vi "Send Message.vi"(8 "error in (no error)":errorcluster, 10 "Message":string, 11 "EUI Events in":refnum<class "EUI Events.lvclass">) -> (0 "error out":errorcluster, 3 "EUI Events out":refnum<class "EUI Events.lvclass">)   [LabVIEW 2016, in "EUI Events.lvclass"]
uses:
  EUI Events.lvclass
  Typedefs/MessageContainer.ctl
  Typedefs/M1M3SupportEUI_TypeDefs.lvlib
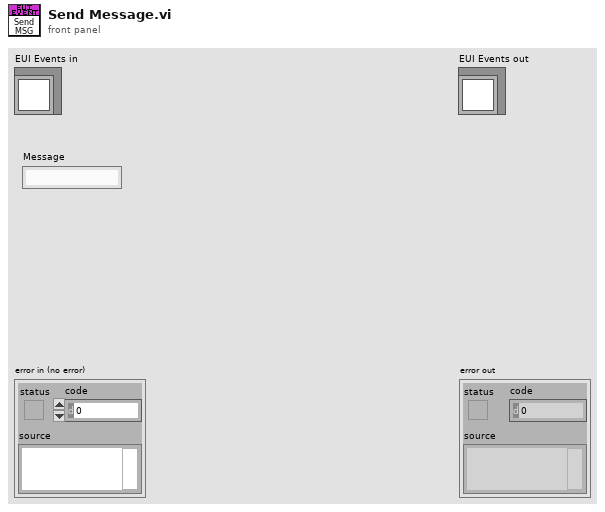
[diagram p1: front panel]
types:
  T1 = typedef "M1M3SupportEUI_TypeDefs.lvlib/MessageContainer.ctl" = cluster{"Message":string, "Time Stamp":timestamp, "Priority":enum16{"Message", "Warning", "Fault", ""}}
  T2 = typedef "M1M3SupportEUI_TypeDefs.lvlib/EUI Events.ctl" = cluster{"Message Event":refnum<user-event>}
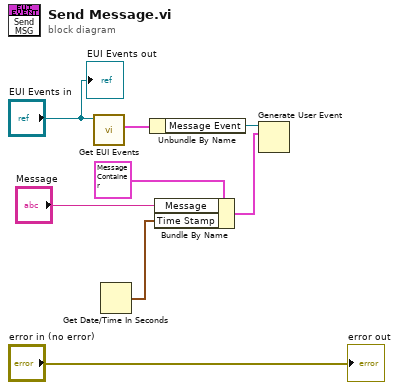
[diagram p0: block diagram]
diagram:
  n1 = call "Get EUI Events.vi"("EUI Events in"="EUI Events in") -> ("EUI Events"=w7:T2)  [unwired: 8 in, 2 out]
  n2 = Get Date/Time In Seconds() -> (seconds since 1Jan1904=w2:timestamp)
  n3 = Unbundle By Name(w7) -> ("Message Event"=w4:refnum<user-event>)
  n4 = Bundle By Name(cluster=T1 {"Message"="", "Time Stamp"=timestamp(0 s since 1904-01-01), "Priority"=enum."Message"} ("event data"), "Message"="Message", "Time Stamp"=w2) -> (w5:T1)
  n5 = Generate User Event(user event=w4, event data cluster=w5) -> ()  [unwired: 2 in, 2 out]
  "error out" <- "error in (no error)"
  "EUI Events out" <- "EUI Events in"
